vi "TCP-IP Read Data Double.vi"(0 "IP address":string="192.168.1.10", 1 "Start Address":string="1028", 9 "No of data regiter read":i32=4, 11 "error in":errorcluster, 12 "remote port or service name":u16=8192) -> (4 "Data regiter":dbl[](array[numeric]), 15 "error out":errorcluster)   [LabVIEW 2015]
panel:
  out "String":string
  out "Array 3":string[](array[string])
  out "Array 2":string[](array[string])
  out "M Intiger":i8[](array[numeric])
  out "substring":string
  out "Array":string[](array[string])
  out "number":dbl[](array[numeric])
  in  "Selector Switch":bool=TRUE
  in  "milliseconds to wait":u32=100
  in  "stop":bool
  out "length":i32
  out "data out":string
  in  "timeout ms":i32=2000
  out "bytes to read":i32
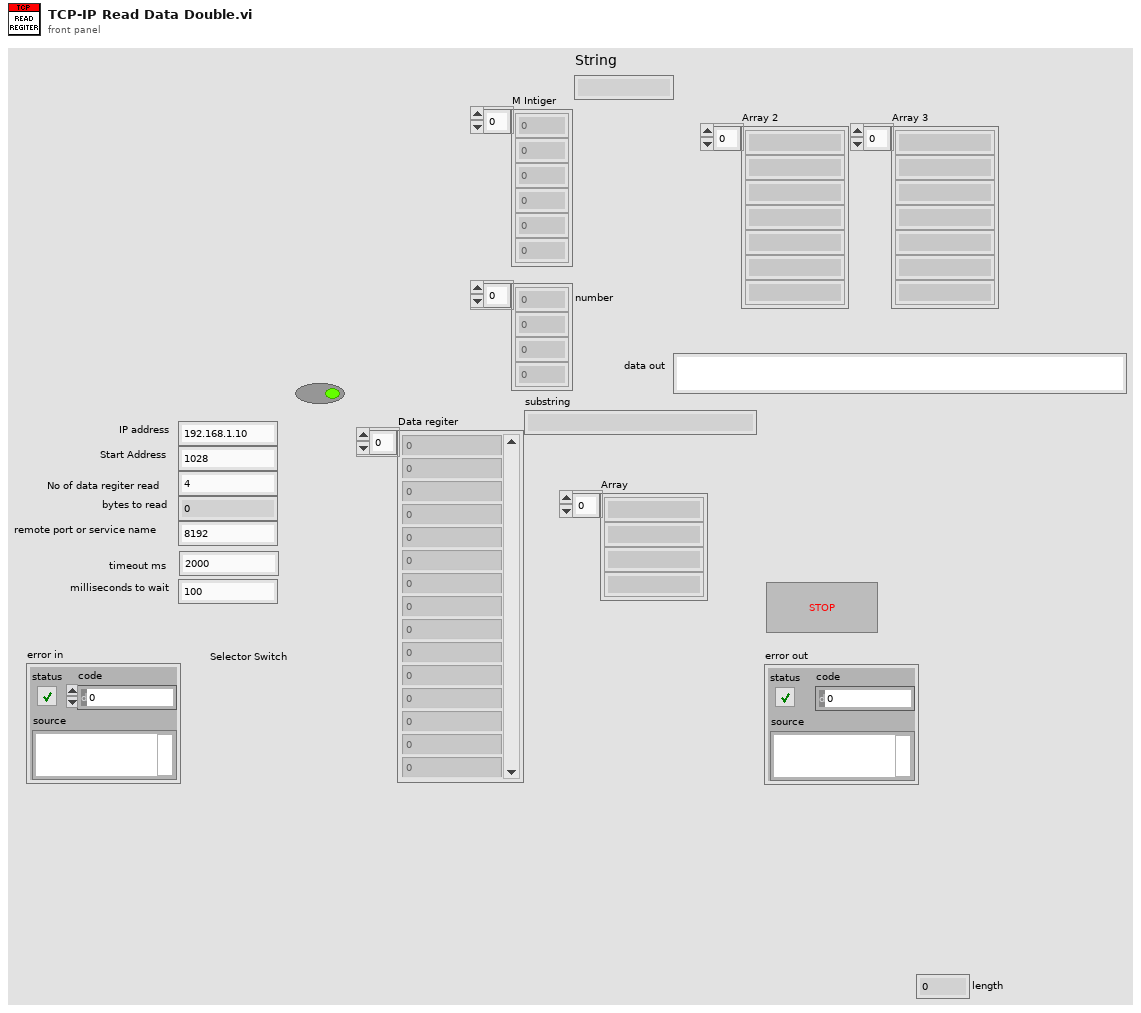
[diagram p1: front panel]
types:
  T1 = enum16{"Standard", "Buffered", "CRLF", "Immediate"}
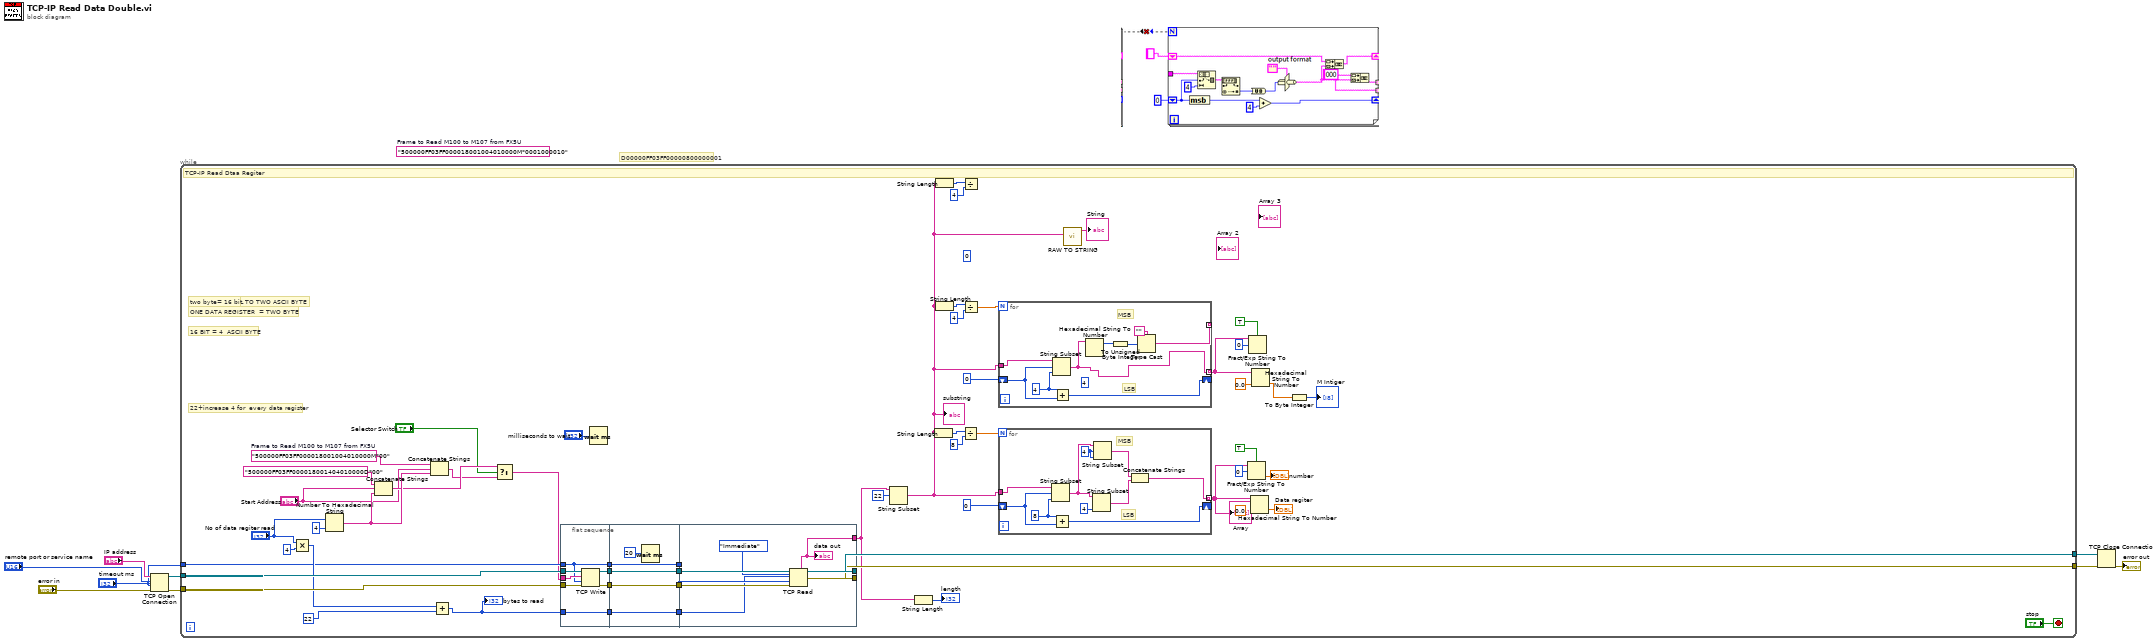
[diagram p0: block diagram]
diagram:
  (unwired) "500000FF03FF000018001004010000M*0001000010"  # Frame to Read M100 to M107 from FX5U
  # "D00000FF03FF00000800000001"
  n1 = TCP Open Connection(address="IP address", remote port or service name="remote port or service name", timeout ms (60000)="timeout ms", error in (no error)="error in") -> (connection ID=w7:refnum<k5>, error out=w6:errorcluster)  [unwired: 1 in]
  n2 = while {
    tunnel: w7 -> [w59]
    tunnel: w6 -> [w58]
    tunnel: "timeout ms" -> [w47]
    tunnel: [w46] -> w3
    tunnel: [w45] -> w2
    stop <- "stop" stop-if-true
    (unwired) 0 ("length (rest)")
    w43 = "500000FF03FF000018001004010000M*00"  # Frame to Read M100 to M107 from FX5U
    # "ONE DATA REGISTER  = TWO BYTE"
    # "ONE BYTE EQUAL TO TWO ASCII BYTE"
    # "16 BIT = 4  ASCII BYTE"
    # "two byte= 16 bit"
    # "22+increase 4 for  every data register"
    # "TCP-IP Read Dtaa Regiter"
    n3 = Multiply(x="No of data regiter read", y=4) -> (x*y=w53:i32)
    n4 = Number To Hexadecimal String(1:i16 4 ("width (-)"), 2:"No of data regiter read") -> (0:w42:string)
    n5 = Concatenate Strings("500000FF03FF000018001404010000D*00", "Start Address", w42) -> (w41:string)
    n6 = Concatenate Strings(w43, "Start Address", w42) -> (w40:string)
    n7 = Add(x=w53, y=22) -> (x+y=w32:i32)
    "bytes to read" <- w32
    n8 = Select(t=w41, s="Selector Switch", f=w40) -> (s? t:f=w38:string)
    n9 = flat-sequence {
      tunnel: w38 -> [w79]
      tunnel: w58 -> [w80]
      tunnel: w59 -> [w81]
      tunnel: w47 -> [w76]
      tunnel: [w78] -> w65
      tunnel: [w77] -> w64
      tunnel: [w76] -> w63
      tunnel: w32 -> [w75]
      tunnel: [w75] -> w30
      tunnel: [w86] -> w62
      tunnel: w65 -> [w86]
      tunnel: [w85] -> w61
      tunnel: w64 -> [w85]
      tunnel: [w83] -> w60
      tunnel: w63 -> [w83]
      tunnel: [w82] -> w31
      tunnel: w30 -> [w82]
      tunnel: [w94] -> w35
      tunnel: w62 -> [w93]
      tunnel: w61 -> [w92]
      tunnel: w60 -> [w91]
      tunnel: [w89] -> w46
      tunnel: [w88] -> w45
      tunnel: w31 -> [w87]
      frame #0 {
        n10 = TCP Write(connection ID=w81, data in=w79, error in (no error)=w80, 9:w76) -> (connection ID out=w78:refnum<k5>, error out=w77:errorcluster)  [unwired: 1 out]
      }
      frame #1 {
        n11 = Wait (ms)(milliseconds to wait=u32 20) -> ()  [unwired: 1 out]
      }
      frame #2 {
        n12 = TCP Read(connection ID=w93, bytes to read=w87, error in (no error)=w92, 7:T1."Immediate" ("mode (standard)"), 9:w91) -> (connection ID out=w89:refnum<k5>, data out=w94:string, error out=w88:errorcluster)
        "data out" <- w94
      }
    }
    n13 = Wait (ms)(milliseconds to wait="milliseconds to wait") -> ()  [unwired: 1 out]
    n14 = String Subset(string=w35, offset (0)=22) -> (substring=w11:string)  [unwired: 1 in]
    "substring" <- w11
    n15 = String Length(string=w35) -> (length=→"length":i32)
    n16 = String Length(string=w11) -> (length=w51:i32)
    n17 = String Length(string=w11) -> (length=w13:i32)
    n18 = String Length(string=w11) -> (length=w16:i32)
    n19 = Divide(x=w51, y=8) -> (x/y=w33:dbl)
    n20 = Divide(x=w13, y=4) -> ()  [unwired: 1 out]
    n21 = Divide(x=w16, y=4) -> (x/y=w19:dbl)
    n22 = for {
      N: w33 -> [_]
      tunnel: w11 -> [w104]
      shift-right: [w103] -> _
      shift-left: 0 ("length (rest)") -> [w102]
      tunnel: [w97] -> w27 mode=indexing
      w99 = 4 ("offset (0)")
      w101 = 8 ("x")
      # "LSB"
      # "MSB"
      n23 = String Subset(string=w104, offset (0)=w102, length (rest)=w101) -> (substring=w98:string)
      n24 = Add(x=w101, y=w102) -> (x+y=w103:i32)
      n25 = String Subset(string=w98, length (rest)=4 ("length (rest)")) -> (substring=w95:string)  [unwired: 1 in]
      n26 = String Subset(string=w98, offset (0)=w99, length (rest)=w99) -> (substring=w96:string)
      n27 = Concatenate Strings(w96, w95) -> (w97:string)
    }
    "Array" <- w27
    n28 = for {
      N: w19 -> [_]
      tunnel: w11 -> [w74]
      shift-right: [w73] -> _
      shift-left: 0 ("length (rest)") -> [w72]
      tunnel: [w70] -> w21 mode=indexing
      tunnel: [w67] -> _ mode=indexing
      (unwired) 4 ("length (rest)")
      w71 = 4 ("x")
      # "LSB"
      # "MSB"
      n29 = String Subset(string=w74, offset (0)=w72, length (rest)=w71) -> (substring=w70:string)
      n30 = Add(x=w71, y=w72) -> (x+y=w73:i32)
      n31 = Hexadecimal String To Number(string=w70) -> (offset past number=w69:i32)  [unwired: 2 in, 1 out]
      n32 = To Unsigned Byte Integer(number=w69) -> (unsigned 8bit integer=w68:u8)
      n33 = Type Cast(type="", x=w68) -> (*(type *) &x=w67:string)
    }
    n34 = call "RAW TO STRING.vi"("data out"=w11) -> ("String"=→"String":string)  [unwired: 10 in]
    n35 = Fract/Exp String To Number(use system decimal point (T)=TRUE, string=w27, offset=0) -> (number=→"number":dbl[])  [unwired: 1 in, 1 out]
    n36 = Fract/Exp String To Number(use system decimal point (T)=TRUE, string=w21, offset=0) -> ()  [unwired: 1 in, 2 out]
    n37 = Hexadecimal String To Number(string=w27, default (0uL)=0.0 ("default (0 U32)")) -> (number=→"Data regiter":dbl[])  [unwired: 1 in, 1 out]
    n38 = Hexadecimal String To Number(string=w21, default (0uL)=0.0 ("default (0 U32)")) -> (number=w15:dbl[])  [unwired: 1 in, 1 out]
    n39 = To Byte Integer(number=w15) -> (8bit integer=→"M Intiger":i8[])
  }
  n40 = TCP Close Connection(connection ID=w3, error in (no error)=w2) -> (error out=→"error out":errorcluster)  [unwired: 1 in, 1 out]
